vi "Rework Count.vi"(8 "error in":errorcluster, 10 "Read /Write":enum16{"Write", "Read"}(ring), 11 "Count For Rework":T1) -> (0 "error out":errorcluster, 3 "data":T1)   [LabVIEW 2015]
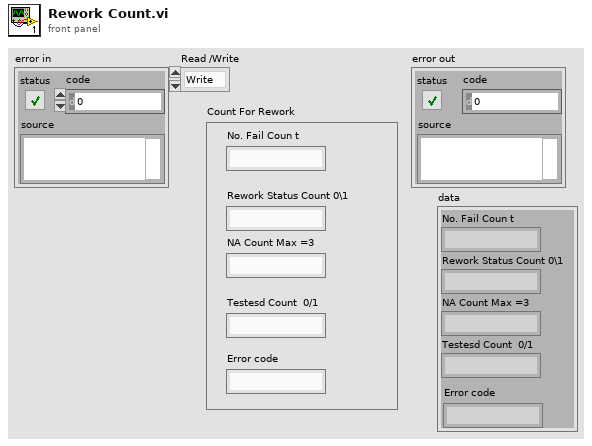
[diagram p1: front panel]
types:
  T1 = cluster{"No. Fail Coun t":string, "Rework Status Count 0\\1":string, "NA Count Max =3 ":string, "Testesd Count  0/1":string, "Error code":string}
  T2 = enum16{"open", "replace", "create", "open or create", "replace or create", "replace or create with confirmation"}
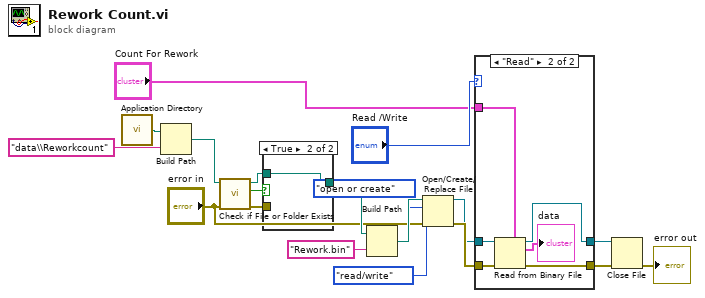
[diagram p0: block diagram]
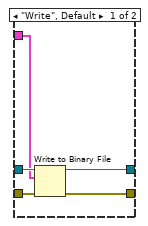
[diagram p2: hidden frame]
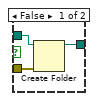
[diagram p3: hidden frame]
diagram:
  n1 = call <vilib>:"Application Directory.vi"() -> ("Application Directory"=w18:path)
  n2 = Build Path(base path=w18, name or relative path="data\\Reworkcount") -> (appended path=w16:path)
  n3 = call <vilib>:"Check if File or Folder Exists.vi"("error in (no error)"="error in", "path"=w16) -> ("error out"=w15:errorcluster, "file or folder exists?"=w14:bool, "dup path"=w17:path)  [unwired: 7 in]
  n4 = case shown="True" w14 {
    tunnel: w17 -> [w22 w23]
    tunnel: [w21 w23] -> w13
    tunnel: w15 -> [w20 _]
    frame False {
      n5 = Create Folder(path (use dialog)=w22, error in=w20) -> (created path=w21:path)  [unwired: 1 in, 2 out]
    }
    frame True {
    }
  }
  n6 = Build Path(base path=w13, name or relative path="Rework.bin") -> (appended path=w6:path)
  n7 = Open/Create/Replace File(file path (use dialog)=w6, error in="error in", operation (0:open)=T2."open or create", access (0:read/write)=enum16{"read/write", "read-only", "write-only"}."read/write") -> (refnum out=w3:refnum<file>, error out=w4:errorcluster)  [unwired: 2 in, 1 out]
  n8 = case shown="\"Read\"" "Read /Write" {
    tunnel: w3 -> [w28 w34]
    tunnel: "Count For Rework" -> [w27 w32]
    tunnel: w4 -> [w26 w33]
    tunnel: [w25 w30] -> w8
    tunnel: [w24 w29] -> w9
    frame "Write", Default {
      n9 = Write to Binary File(file (use dialog)=w28, data=w27, error in=w26) -> (refnum out=w24:refnum<file>, error out=w25:errorcluster)  [unwired: 3 in, 1 out]
    }
    frame "Read" {
      n10 = Read from Binary File(5:w32, 8:w33, 11:w34) -> (0:w30:errorcluster, 2:→"data":T1, 3:w29:refnum<file>)  [unwired: 3 in, 1 out]
    }
  }
  n11 = Close File(refnum=w9, error in=w8) -> (error out=→"error out":errorcluster)  [unwired: 1 out]
